vi "XIPIN_Linear_Algebra_Toolkit_1_0.vi"   [LabVIEW 2017]
doc: "The Xilinx LogiCORE (TM) IP Linear Algebra Toolkit (LAT) v1.0 implements the basic Matrix operations, namely, Matrix-Matrix Addition, Subtraction, Matrix-Scalar Multiplication and Matrix-Matrix Multiplication. This IP provides flexible and optimized building blocks to the customer for developing complex composite functions for various signal and data processing applications.\n------------------------------------\n<b>Need License</b> : No\n<b>Interface</b> : AXI4-Stream"
uses:
  <vilib>/rvi/XilinxIP/XIPIN_XNode/niFpgaXIPIN.xnode
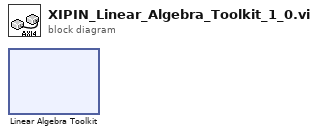
[diagram p0: block diagram]
diagram:
  n1 = xnode ("Linear Algebra Toolkit")() -> ()
